vi "populateBroadcastSetForceFrame.vi"(8 "error in (no error)":errorcluster, 10 "FixedFrameBuilder in":refnum<class "FixedFrameBuilder.lvclass">, 11 "FAILC in":refnum<class "FAILC.lvclass">) -> (0 "error out":errorcluster, 2 "FixedFrameBuilder out":refnum<class "FixedFrameBuilder.lvclass">, 3 "FAILC out":refnum<class "FAILC.lvclass">)   [LabVIEW 2016, in "RTFAILC.lvlib" / "FAILC.lvclass"]
uses:
  FAILC.lvclass
  D:/Code/ts_FAMT/Common_RT_ILC/ILC/ILC.lvclass
  Common_RT_Modbus/FixedFrameBuilder/FixedFrameBuilder.lvclass
  FAILC.lvclass/FAILC.ctl
  Common_RT_ILC/ILC/ILC.lvclass/ILC.ctl
  Common_RT_ILC/ILC/ILC.lvclass
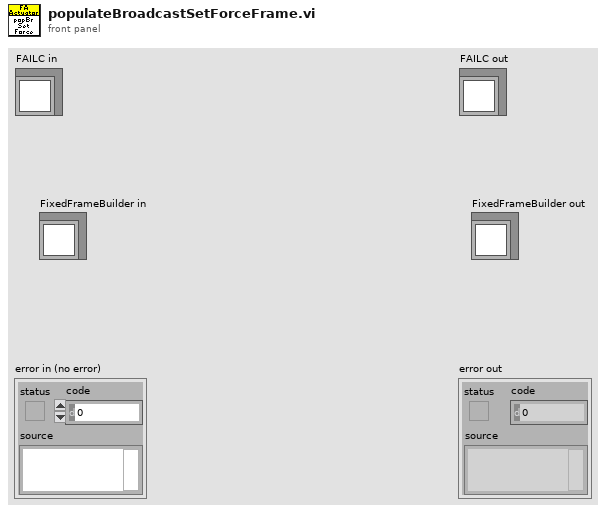
[diagram p1: front panel]
types:
  T1 = typedef "RTILC.lvlib/ILCData.ctl" = cluster{"Constants":T2, "Command":T3, "Telemetry":T5, "Responses":T6}
  T2 = typedef "RTILC.lvlib/ILCConstants.ctl" = cluster{"Subnet":u8, "Address":u8}
  T3 = typedef "RTILC.lvlib/ILCCommand.ctl" = cluster{"ILCMode":u16, "TemporaryAddress":u8, "ADCScanRate":T4, "ADCChannel":u8, "ADCOffset":sgl, "ADCSensitivity":sgl}
  T4 = typedef "RTILC.lvlib/ILCScanRates.ctl" = u8
  T5 = typedef "RTILC.lvlib/ILCTelemetry.ctl" = cluster{"UniqueID":u64, "FirmwareType":u8, "NetworkNodeType":u8, "ILCOption":u8, "NetworkNodeOption":u8, "MajorRevision":u8, "MinorRevision":u8, "FirmwareName":string, "ILCMode":u16, "MajorFault":bool, "MinorFault":bool, "FaultOverride":bool, "UniqueIDCRCMismatch":bool, "AppTypeNodeTypeMismatch":bool, "AppMissing":bool, "AppCRCMismatch":bool, "TEDSNotFound":bool, "TEDS1Mismatch":bool, "TEDS2Mismatch":bool, "WatchdogResetDetected":bool, "BrownoutDetected":bool, "EventTrapResetDetected":bool, "TemporaryAddress":u8, "ADCScanRate":T4, "DAC1":u16, "DAC2":u16, "DAC3":u16, "DAC4":u16, "MainADCCalibrationK":sgl[], "MainSensorOffset":sgl[], "MainSensorSensitivity":sgl[], "BackupADCCalibrationK":sgl[], "BackupSensorOffset":sgl[], "BackupSensorSensitivity":sgl[]}
  T6 = typedef "RTILC.lvlib/ILCResponses.ctl" = cluster{"ReportServerID":T7, "ReportServerStatus":T7, "ILCMode":T7, "SetTemporaryAddress":T7, "Reset":T7, "ADCScanRate":T7, "ADCOffsetSensitivity":T7, "ReadDAC":T7, "ReadCalibration":T7}
  T7 = typedef "RTModbus.lvlib/ExceptionCodes.ctl" = u16
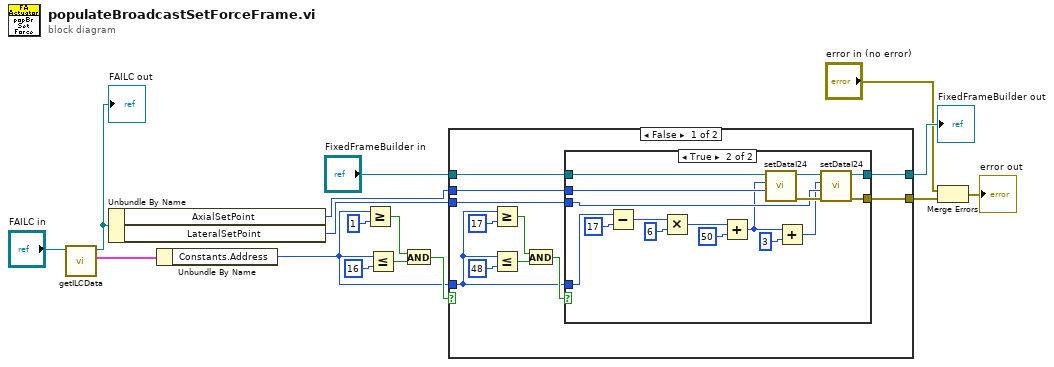
[diagram p0: block diagram]
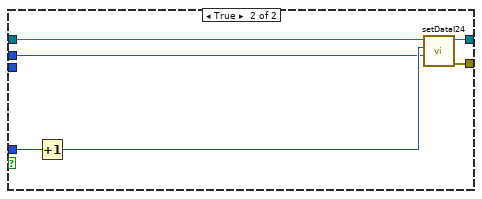
[diagram p3: hidden frame]
diagram:
  n1 = call "getILCData.vi"("ILC in"="FAILC in") -> ("ILCData"=w12:T1, "ILC out"=w2:refnum<class "FAILC.lvclass">)  [unwired: 9 in]
  "FAILC out" <- w2
  n2 = Unbundle By Name(w2) -> ("AxialSetPoint"=w7:i32, "LateralSetPoint"=w1:i32)
  n3 = Unbundle By Name(w12) -> ("Constants.Address"=w8:u8)
  n4 = Greater Or Equal?(x=w8, y=u8 1) -> (x >= y?=w16:bool)
  n5 = Less Or Equal?(x=w8, y=u8 16) -> (x <= y?=w15:bool)
  n6 = And(x=w16, y=w15) -> (x .and. y?=w14:bool)
  n7 = case shown="False" w14 {
    tunnel: "FixedFrameBuilder in" -> [w22 w50]
    tunnel: w8 -> [w17 w49]
    tunnel: w7 -> [w19 w47]
    tunnel: [w21 w46] -> w6
    tunnel: [w20 w45] -> w5
    tunnel: w1 -> [w18 _]
    frame False {
      n8 = Greater Or Equal?(x=w17, y=u8 17) -> (x >= y?=w26:bool)
      n9 = Less Or Equal?(x=w17, y=u8 48) -> (x <= y?=w27:bool)
      n10 = And(x=w26, y=w27) -> (x .and. y?=w25:bool)
      n11 = case shown="True" w25 {
        tunnel: w22 -> [w28 w44]
        tunnel: [w28 w42] -> w21
        tunnel: [_ w40] -> w20
        tunnel: w19 -> [_ w39]
        tunnel: w18 -> [_ w38]
        tunnel: w17 -> [_ w35]
        frame False {
        }
        frame True {
          n12 = Subtract(x=w35, y=u8 17) -> (x-y=w36:u8)
          n13 = Multiply(x=w36, y=u8 6) -> (x*y=w32:u8)
          n14 = Add(x=w32, y=u8 50) -> (x+y=w31:u8)
          n15 = call "setDataI24.vi"("Data"=w39, "Index"=w31, "FixedFrameBuilder in"=w44) -> ("error out"=w41:errorcluster, "FixedFrameBuilder out"=w43:refnum<class "FixedFrameBuilder.lvclass">)  [unwired: 7 in]
          n16 = Add(x=w31, y=u8 3) -> (x+y=w29:u8)
          n17 = call "setDataI24.vi"("error in (no error)"=w41, "Data"=w38, "Index"=w29, "FixedFrameBuilder in"=w43) -> ("error out"=w40:errorcluster, "FixedFrameBuilder out"=w42:refnum<class "FixedFrameBuilder.lvclass">)  [unwired: 6 in]
        }
      }
    }
    frame True {
      n18 = Increment(x=w49) -> (x+1=w48:u8)
      n19 = call "setDataI24.vi"("Data"=w47, "Index"=w48, "FixedFrameBuilder in"=w50) -> ("error out"=w45:errorcluster, "FixedFrameBuilder out"=w46:refnum<class "FixedFrameBuilder.lvclass">)  [unwired: 7 in]
    }
  }
  "FixedFrameBuilder out" <- w6
  n20 = Merge Errors("error in (no error)", w5) -> (→"error out":errorcluster)
